vi "U6 Pin Configuration.vi"(4 "Enable Counter1":bool, 6 "Enable Counter0":bool, 8 "error in":errorcluster, 10 "Number of Timers Enabled":u8, 11 "Handle In":i32) -> (0 "error out":errorcluster, 3 "Handle Out":i32)   [LabVIEW 2021]
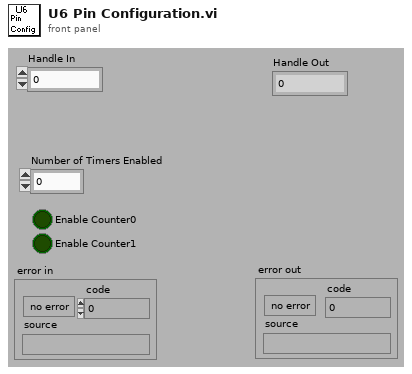
[diagram p1: front panel]
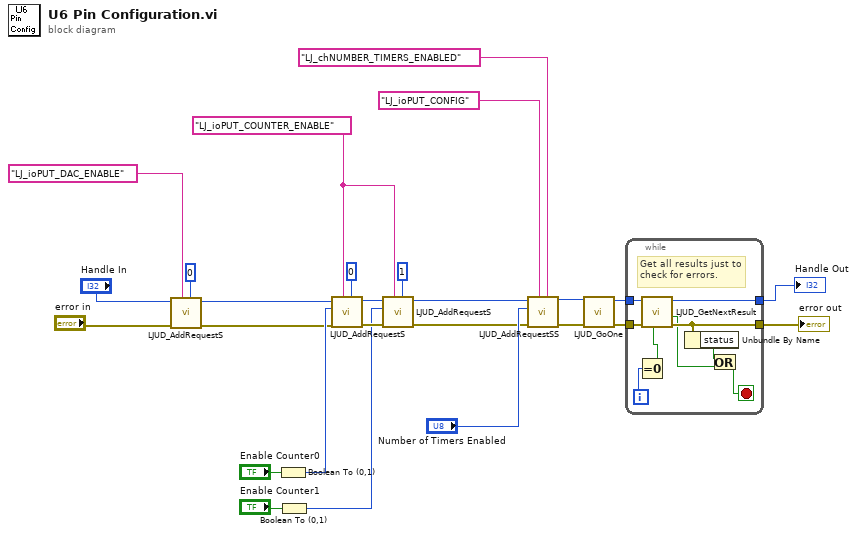
[diagram p0: block diagram]
diagram:
  w17 = "LJ_ioPUT_COUNTER_ENABLE" ("Channel")
  n1 = call "LJUD_AddRequestS.vi"("Channel"=0, "IOType"="LJ_ioPUT_DAC_ENABLE" ("Channel"), "error in"="error in", "Handle In"="Handle In") -> ("error out"=w7:errorcluster, "Handle Out"=w6:i32)  [unwired: 6 in]
  n2 = Boolean To (0,1)(Boolean="Enable Counter0") -> (0, 1=w11:i16)
  n3 = Boolean To (0,1)(Boolean="Enable Counter1") -> (0, 1=w10:i16)
  n4 = call "LJUD_AddRequestS.vi"("Channel"=0, "IOType"=w17, "error in"=w7, "Value"=w11, "Handle In"=w6) -> ("error out"=w19:errorcluster, "Handle Out"=w18:i32)  [unwired: 5 in]
  n5 = call "LJUD_AddRequestS.vi"("Channel"=1, "IOType"=w17, "error in"=w19, "Value"=w10, "Handle In"=w18) -> ("error out"=w1:errorcluster, "Handle Out"=w2:i32)  [unwired: 5 in]
  n6 = call "LJUD_AddRequestSS.vi"("Channel"="LJ_chNUMBER_TIMERS_ENABLED", "IOType"="LJ_ioPUT_CONFIG", "error in"=w1, "Value"="Number of Timers Enabled", "Handle In"=w2) -> ("error out"=w26:errorcluster, "Handle Out"=w25:i32)  [unwired: 5 in]
  n7 = call "LJUD_GoOne.vi"("error in"=w26, "Handle In"=w25) -> ("error out"=w24:errorcluster, "Handle Out"=w23:i32)  [unwired: 8 in]
  n8 = while {
    tunnel: w24 -> [w33]
    tunnel: w23 -> [w32]
    tunnel: [w31] -> w20
    tunnel: [w29] -> w12
    i -> [w28]
    stop <- w35 stop-if-true
    # "Get all results just to\ncheck for errors."
    n9 = Equal To 0?(x=w28) -> (x = 0?=w34:bool)
    n10 = call "LJUD_GetNextResult.vi"("GetFirst"=w34, "error in"=w33, "Handle In"=w32) -> ("error out"=w31:errorcluster, "LJE_NO_MORE_DATA_AVAILABLE"=w27:bool, "Handle Out"=w29:i32)  [unwired: 3 in, 3 out]
    n11 = Unbundle By Name(w31) -> ("status"=w30:bool)
    n12 = Or(x=w30, y=w27) -> (x .or. y?=w35:bool)
  }
  "error out" <- w20
  "Handle Out" <- w12
